vi "Admin.vi"() -> ()   [LabVIEW 2016]
uses:
  <vilib>/httpClient/LabVIEWHTTPClient.lvlib
panel:
  out "new picture":picture
  in  "String 2":string
  in  "String":string
  in  "?":bool
  # "Administration"
  # "Username : \n\n   \n    Password :"
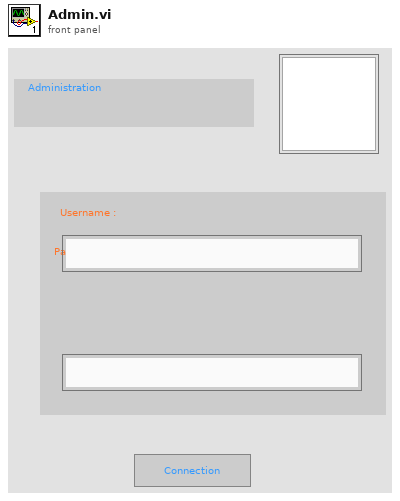
[diagram p1: front panel]
types:
  T1 = typedef "imagedata.ctl" = cluster{"image type":i32, "image depth":i32, "image":u8[], "mask":u8[], "colors":u32[], "Rectangle":cluster{"left":i16, "top":i16, "right":i16, "bottom":i16}}
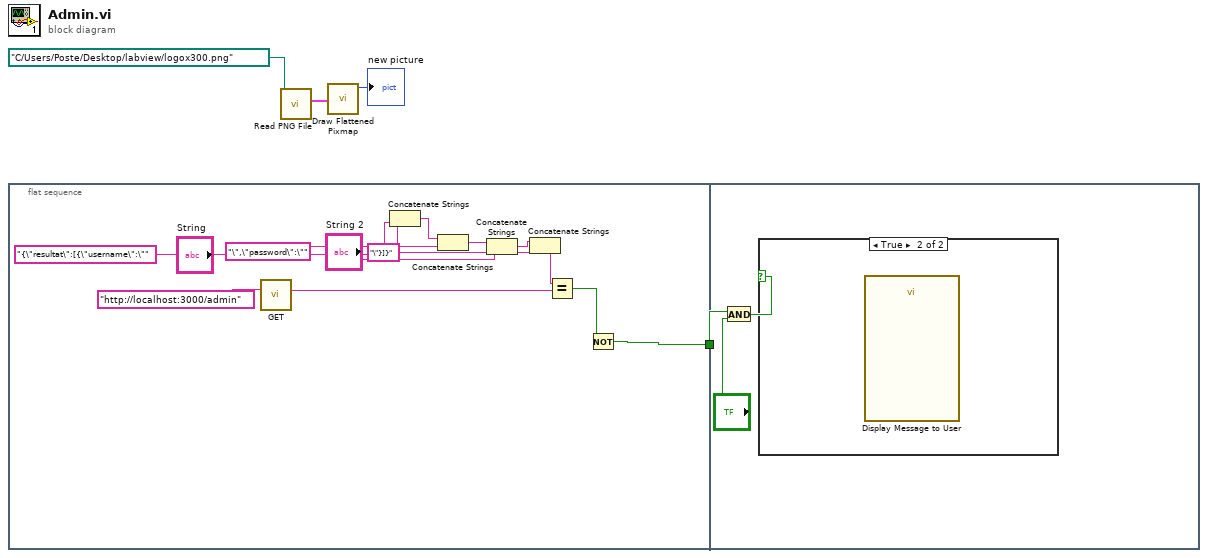
[diagram p0: block diagram]
diagram:
  n1 = flat-sequence {
    tunnel: [w5] -> w4
    tunnel: w4 -> [w18]
    frame #0 {
      n2 = call <vilib>:"GET.vi"("url"="http://localhost:3000/admin") -> ("body"=w13:string)  [unwired: 11 in, 3 out]
      n3 = Concatenate Strings("{\"resultat\":[{\"username\":\"", "String") -> (w14:string)
      n4 = Concatenate Strings(w14, "\",\"password\":\"") -> (w11:string)
      n5 = Concatenate Strings(w11, "String 2") -> (w9:string)
      n6 = Concatenate Strings(w9, "\"}]}") -> (w7:string)
      n7 = Equal?(x=w7, y=w13) -> (x = y?=w6:bool)
      n8 = Not(x=w6) -> (.not. x?=w5:bool)
    }
    frame #1 {
      n9 = And(x=w18, y="?") -> (x .and. y?=w19:bool)
      n10 = case shown="True" w19 {
        frame False {
        }
        frame True {
          n11 = call "Display Message to User"() -> ()  [unwired: 10 in, 2 out]
        }
      }
    }
  }
  n12 = call <vilib>:"Read PNG File.vi"("path to PNG file"=path "C:/Users/Poste/Desktop/labview/logox300.png") -> ("image data"=w2:T1)  [unwired: 8 in, 2 out]
  n13 = call <vilib>:"Draw Flattened Pixmap.vi"("image data"=w2) -> ("new picture"=→"new picture":picture)  [unwired: 8 in]
